vi "Password base system.vi"() -> ()   [LabVIEW 2018]
panel:
  out "RESULT":string
  in  "PASSWORD":string
  in  "USERNAME":string
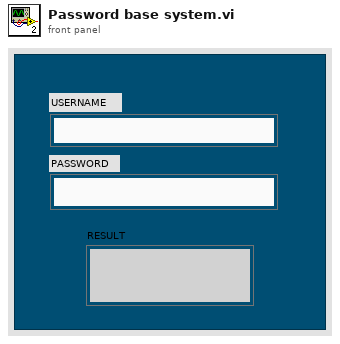
[diagram p1: front panel]
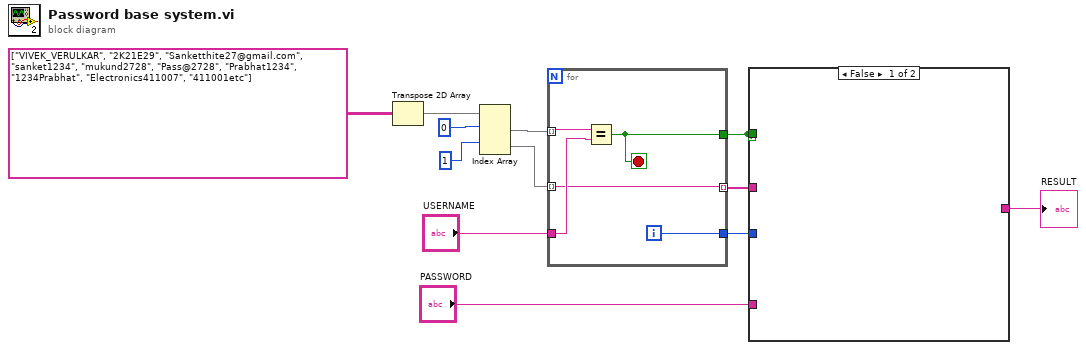
[diagram p0: block diagram]
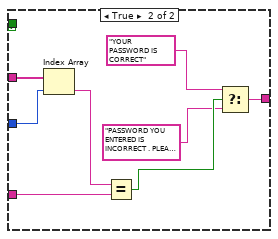
[diagram p2: hidden frame]
diagram:
  n1 = Transpose 2D Array(2D array=string[][] [["VIVEK_VERULKAR", "2K21E29"], ["Sanketthite27@gmail.com", "sanket1234"], ["mukund2728", "Pass@2728"], ["Prabhat1234", "1234Prabhat"], ["Electronics411007", "411001etc"]]) -> (transposed array=w11:string[][])
  n2 = Index Array "Index Array"(array=w11, index (row) #1=0 ("index (row)"), index (row) #2=1 ("index (row)")) -> (element #1=w8:string[], element #2=w5:string[])  [unwired: 2 in]
  n3 = for {
    tunnel: w8 -> [w17] mode=indexing
    tunnel: "USERNAME" -> [w16]
    tunnel: [w15] -> w6 mode=indexing
    tunnel: w5 -> [w15] mode=indexing
    tunnel: [w14] -> w4
    tunnel: [w13] -> w2
    i -> [w14]
    stop <- w13 stop-if-true
    n4 = Equal?(x=w17, y=w16) -> (x = y?=w13:bool)
  }
  n5 = case shown="False" w2 {
    tunnel: w6 -> [_ w25]
    tunnel: w4 -> [_ w24]
    tunnel: "PASSWORD" -> [_ w23]
    tunnel: w2 -> [_ _]
    tunnel: [_ w20] -> w1
    frame False {
    }
    frame True {
      n6 = Index Array "Index Array"(array=w25, index=w24) -> (element=w22:string)
      n7 = Equal?(x=w22, y=w23) -> (x = y?=w21:bool)
      n8 = Select(t="YOUR PASSWORD IS CORRECT" ("f"), s=w21, f="PASSWORD YOU ENTERED IS INCORRECT . PLEASE TRY AGAIN.") -> (s? t:f=w20:string)
    }
  }
  "RESULT" <- w1
